vi "Flash LED.vi"(0 "Boolean in":refnum<vi>, 7 "milliseconds to wait":dbl=1000.0, 11 "error in (no error)":errorcluster) -> (4 "Boolean out":refnum<vi>, 15 "error out":errorcluster)   [LabVIEW 2020]
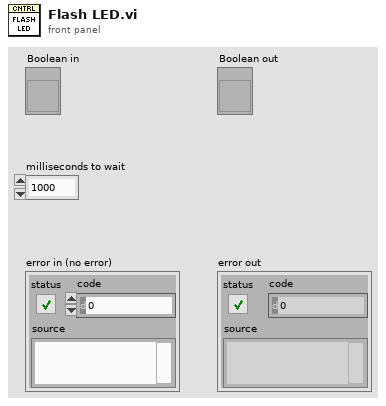
[diagram p1: front panel]
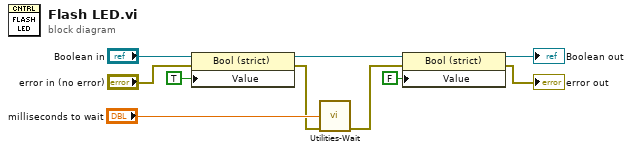
[diagram p0: block diagram]
diagram:
  n1 = property class="Bool (strict)"(reference="Boolean in", error in="error in (no error)", "Value"=TRUE) -> (reference out=w6:refnum<vi>, error out=w3:errorcluster)
  n2 = call "Utilities-Wait.vi"("milliseconds to wait"="milliseconds to wait", "error in (no error)"=w3) -> ("error out"=w5:errorcluster)  [unwired: 13 in]
  n3 = property class="Bool (strict)"(reference=w6, error in=w5, "Value"=FALSE) -> (reference out=→"Boolean out":refnum<vi>, error out=→"error out":errorcluster)
